vi "DistillTitle.vi"(7 "Plot Summary in":string[][](array[string]), 8 "Show Channels with range of Values?":bool, 10 "Indices to include in Page Title":i32[](array[numeric]), 11 "String in":string) -> (3 "String out":string, 4 "AvailableVariables":string[](array[string]))   [LabVIEW 2021]
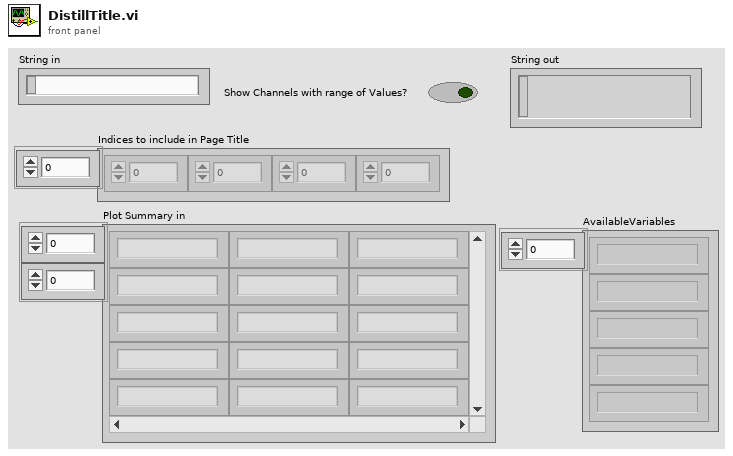
[diagram p1: front panel]
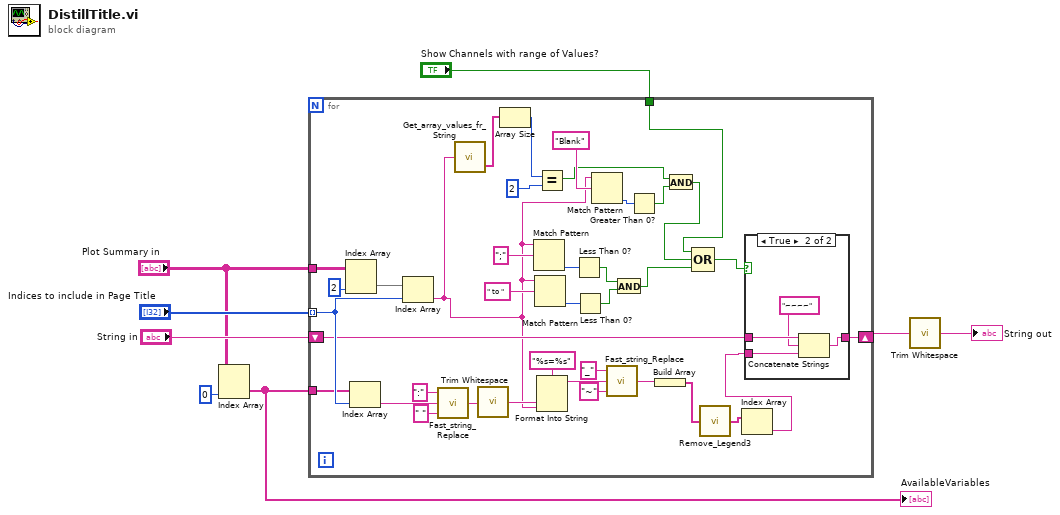
[diagram p0: block diagram]
diagram:
  n1 = Index Array(array="Plot Summary in", index (col)=0 ("disabled index (col)")) -> (element=w5:string[])  [unwired: 1 in]
  "AvailableVariables" <- w5
  n2 = for {
    tunnel: "Indices to include in Page Title" -> [w45] mode=indexing
    tunnel: "Plot Summary in" -> [w46]
    shift-right: [w36] -> w6
    shift-left: "String in" -> [w37]
    tunnel: w5 -> [w34]
    tunnel: "Show Channels with range of Values?" -> [w16]
    n3 = Index Array(array=w46, index (col)=2 ("index (row)")) -> (element=w44:string[])  [unwired: 1 in]
    n4 = Index Array(array=w34, index=w45) -> (element=w40:string)
    n5 = Index Array(array=w44, index=w45) -> (element=w14:string)
    n6 = call "Fast_string_Replace.vi"("Replace match with:"=" ", "Input String"=w40, "regular expression"=":") -> ("Output String"=w39:string)  [unwired: 2 out]
    n7 = call "Get_array_values_fr_String.vi"("String Value"=w14) -> ("String array"=w13:string[])  [unwired: 1 out]
    n8 = call <vilib>:"Trim Whitespace.vi"("string"=w39) -> ("trimmed string"=w38:string)  [unwired: 1 in]
    n9 = Array Size(array=w13) -> (size(s)=w23:i32)
    n10 = Match Pattern(string=w14, regular expression=";") -> (offset past match=w29:i32)  [unwired: 4 out]
    n11 = Match Pattern(string=w14, regular expression=" to ") -> (offset past match=w30:i32)  [unwired: 4 out]
    n12 = Equal?(x=w23, y=2) -> (x = y?=w17:bool)
    n13 = Format Into String(format string="%s=%s", w38, w14) -> (resulting string=w26:string)  [unwired: 2 in, 1 out]
    n14 = Less Than 0?(x=w29) -> (x < 0?=w21:bool)
    n15 = Less Than 0?(x=w30) -> (x < 0?=w31:bool)
    n16 = Match Pattern(string=w14, regular expression="Blank" ("x")) -> (offset past match=w19:i32)  [unwired: 4 out]
    n17 = call "Fast_string_Replace.vi"("Replace match with:"="~", "Input String"=w26, "regular expression"="_") -> ("Output String"=w9:string)  [unwired: 2 out]
    n18 = And(x=w21, y=w31) -> (x .and. y?=w24:bool)
    n19 = Greater Than 0?(x=w19) -> (x > 0?=w18:bool)
    n20 = Build Array(w9) -> (w12:string[])
    n21 = And(x=w17, y=w18) -> (x .and. y?=w15:bool)
    n22 = Compound Arithmetic op=OR(w16, w15, w24) -> (w25:bool)
    n23 = call "Remove_Legend3.vi"("Ordinate Strings"=w12) -> ("Array"=w11:string[])
    n24 = Index Array(array=w11) -> (element=w10:string)  [unwired: 1 in]
    n25 = case shown="True" w25 {
      tunnel: w37 -> [w47 w51]
      tunnel: [w47 w50] -> w36
      tunnel: w10 -> [_ w49]
      frame False {
      }
      frame True {
        n26 = Concatenate Strings(w51, "~~~~" ("string"), w49) -> (w50:string)
      }
    }
  }
  n27 = call <vilib>:"Trim Whitespace.vi"("string"=w6) -> ("trimmed string"=→"String out":string)  [unwired: 1 in]
